vi "Write session.vi"(8 "error in (no error)":errorcluster, 10 "session in":refnum<k21>, 11 "SLSC Switch in":refnum<class "SLSC Switch.lvclass">) -> (0 "error out":errorcluster, 3 "SLSC Switch out":refnum<class "SLSC Switch.lvclass">)   [LabVIEW 2015, in "SLSC Switch.lvclass"]
uses:
  SLSC Switch.lvclass
  SLSC Switch.lvclass/SLSC Switch.ctl
  <vilib>/SLSC/Close Session.vi
  <vilib>/SLSC/SLSC.lvlib
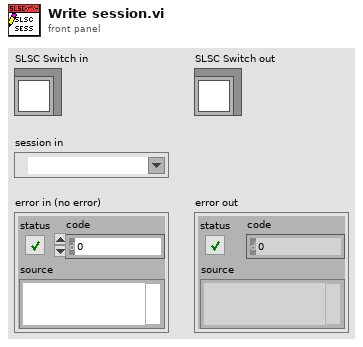
[diagram p1: front panel]
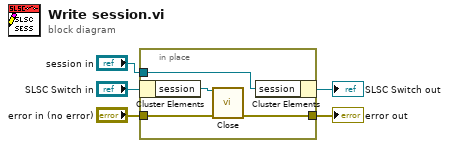
[diagram p0: block diagram]
diagram:
  n1 = in-place {
    in-place-border: "session in" -> [w8]
    in-place-border: "error in (no error)" -> [w7]
    in-place-border: [w6] -> w2
    n2 = in-place-cluster #1("SLSC Switch in") -> ("session"=w9:refnum<k21>)
    n3 = call-poly <vilib>:"Close.vi"("session in"=w9, "error in (no error)"=w7) -> ("error out"=w6:errorcluster)  [unwired: 13 in]
    n4 = in-place-cluster #1("session"=w8) -> (→"SLSC Switch out":refnum<class "SLSC Switch.lvclass">)
  }
  "error out" <- w2
